vi "Buzzer(SubVI).vi"(8 "error in (no error)":errorcluster, 10 "LINX Resource in":T1, 11 "Buzzer Channel":u8) -> (0 "error out":errorcluster, 3 "LINX Resource out":T1)   [LabVIEW 2020]
uses:
  <vilib>/MakerHub/LINX/Private/Type Defs/LINX Ref.ctl
  <vilib>/MakerHub/LINX/Private/Type Defs/Platform.ctl
  <vilib>/MakerHub/LINX/Private/Type Defs/Interface.ctl
  <vilib>/MakerHub/LINX/Private/Device/Type Defs/LINX Device Config.ctl
  <vilib>/MakerHub/LINX/Private/Device/Type Defs/TCP Config.ctl
  <vilib>/MakerHub/LINX/Private/Device/Type Defs/Channels.ctl
  <vilib>/MakerHub/LINX/LMH-LINX.lvlib
  <vilib>/MakerHub/LINX/Private/Device/Device.lvlib
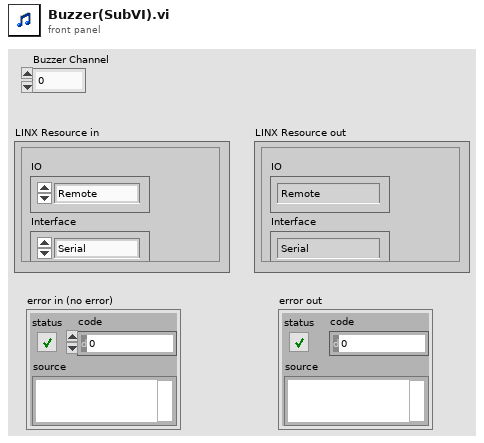
[diagram p1: front panel]
types:
  T1 = typedef "LMH-LINX.lvlib/LINX Ref.ctl" = cluster{"IO":T2, "Interface":T3, "LINX Device Config":T4}
  T2 = typedef "LMH-LINX.lvlib/Platform.ctl" = enum16{"Remote", "Local"}
  T3 = typedef "LMH-LINX.lvlib/Interface.ctl" = enum16{"Serial", "TCP"}
  T4 = typedef "LMH-LINX.lvlib/Device.lvlib/LINX Device Config.ctl" = cluster{"Interface":T3, "COM Port":refnum<visa-resource-name>, "TCP Configuration":T5, "Device Family":u8, "Device ID":u8, "Device Name":string, "TCP Ref":refnum<k5>, "Channels":T6}
  T5 = typedef "LMH-LINX.lvlib/Device.lvlib/TCP Config.ctl" = cluster{"IP Address":string, "Port":u16}
  T6 = typedef "LMH-LINX.lvlib/Channels.ctl" = cluster{"DI":u8[], "DO":u8[], "AI":u8[], "AO":u8[], "PWM":u8[], "QE":u8[], "UART":u8[], "I2C 2":u8[], "SPI":u8[], "CAN":u8[], "Servo":u8[], "AI Ref (V)":dbl, "AI Resolution (Bits)":u8, "AO Ref (V)":dbl, "AO Resolution (Bits)":u8}
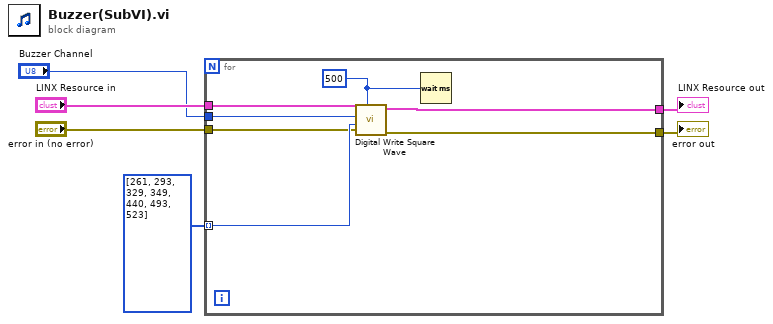
[diagram p0: block diagram]
diagram:
  n1 = for {
    tunnel: i32[] [261, 293, 329, 349, 440, 493, 523] -> [w13] mode=indexing
    tunnel: "Buzzer Channel" -> [w12]
    tunnel: "LINX Resource in" -> [w11]
    tunnel: "error in (no error)" -> [w10]
    tunnel: [w8] -> w5
    tunnel: [w7] -> w6
    w9 = u32 500 ("Duration (ms)")
    n2 = call <vilib>:"Digital Write Square Wave.vi"("Duration (ms)"=w9, "Error In"=w10, "Frequency (Hz)"=w13, "Channel"=w12, "LINX Resource"=w11) -> ("Error Out"=w7:errorcluster, "LINX Resource"=w8:T1)  [unwired: 5 in]
    n3 = Wait (ms)(milliseconds to wait=w9) -> ()  [unwired: 1 out]
  }
  "error out" <- w6
  "LINX Resource out" <- w5
